vi "FTW-JSON-Object-GetElements-Bool.vi"(0 "JSON Object":refnum<class "FTW-JSON.lvclass">, 5 "Keys":string[](array[string]), 11 "error in":errorcluster) -> (4 "JSON Object out":refnum<class "FTW-JSON.lvclass">, 6 "Values":bool[](array[boolean]), 8 "All Found?":bool, 10 "Which Found?":bool[](array[boolean]), 15 "error out":errorcluster)   [LabVIEW 2013, in "FTW-JSON.lvclass"]
uses:
  FTW-JSON.lvclass
  FTW-JSON.lvclass/FTW-JSON.ctl
  FTW-JSON-Type.ctl
panel:
  # "Inputs"
  # "Outputs"
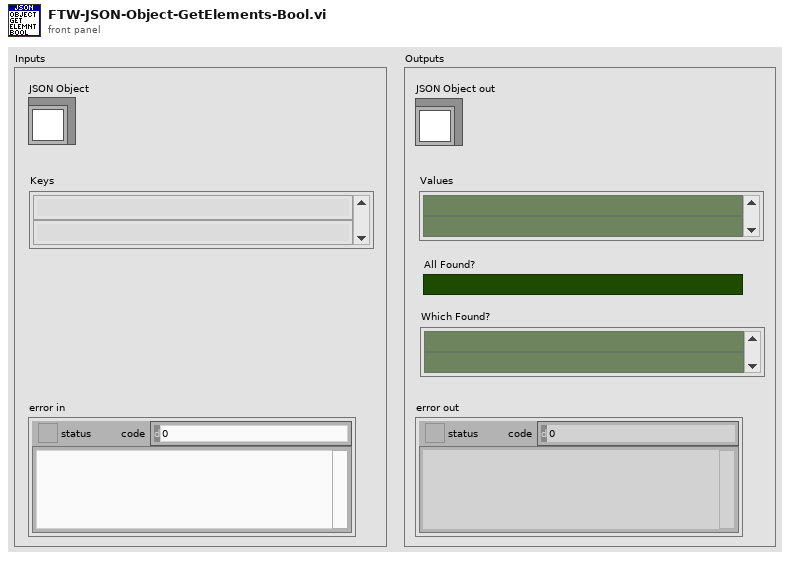
[diagram p1: front panel]
types:
  T1 = typedef "FTW-JSON-Type.ctl" = enum16{"Object", "Array", "String", "Integer", "Floating Point", "true", "false", "null", "undefined"}
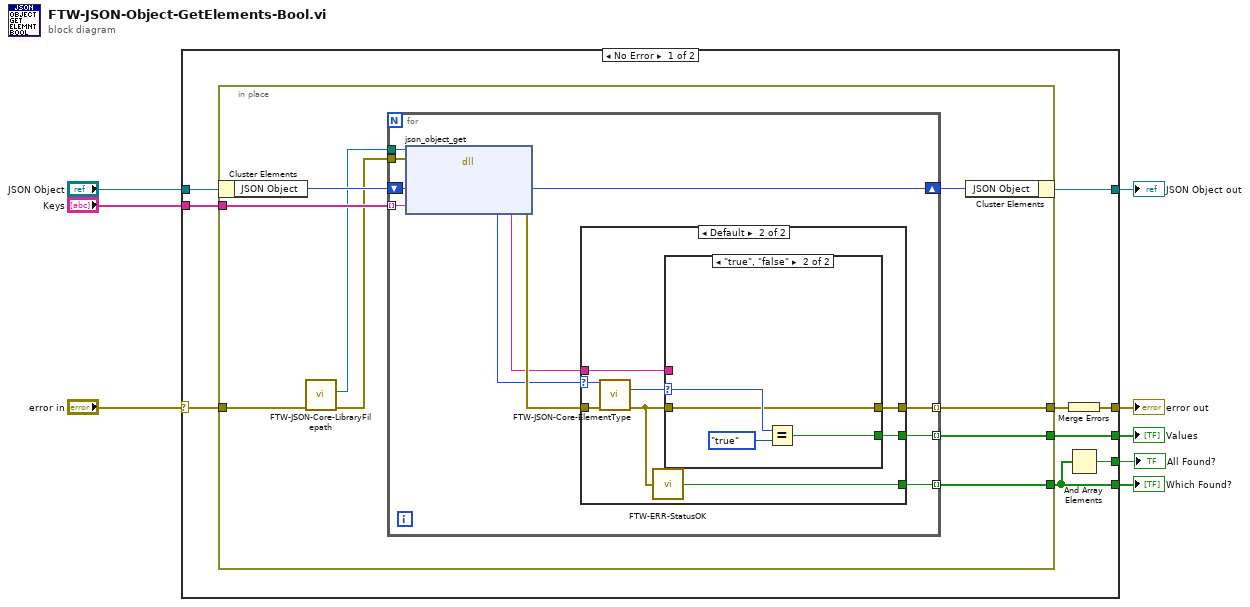
[diagram p0: block diagram]
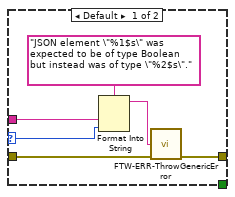
[diagram p3: hidden frame]
diagram:
  n1 = case shown="No Error" "error in" {
    selector: "error in" -> [w17 w58]
    tunnel: [w11 w58] -> w8
    tunnel: [w15 w57] -> w6
    tunnel: "JSON Object" -> [w16 w57]
    tunnel: "Keys" -> [w14 _]
    tunnel: [w12 _] -> w3
    tunnel: [w10 _] -> w2
    tunnel: [w9 _] -> w1
    frame No Error {
      n2 = in-place {
        in-place-border: w17 -> [w26]
        in-place-border: w14 -> [w24]
        in-place-border: [w21] -> w13
        in-place-border: [w20] -> w12
        in-place-border: [w18] -> w10
        n3 = in-place-cluster #1(w16) -> ("JSON Object"=w25:i64)
        n4 = call "FTW-JSON-Core-LibraryFilepath.vi"("error in"=w26) -> ("error out"=w23:errorcluster, "JSON Library Filepath"=w22:path)  [unwired: 9 in]
        n5 = for {
          tunnel: w24 -> [w36] mode=indexing
          tunnel: w23 -> [w35]
          tunnel: w22 -> [w34]
          tunnel: [w32] -> w21 mode=indexing
          tunnel: [w31] -> w20 mode=indexing
          tunnel: [w28] -> w18 mode=indexing
          shift-right: [w29] -> w19
          shift-left: w25 -> [w37]
          n6 = dll-call lib="?" fn="json_object_get"(path in=w34, error in=w35, "JSON Object Pointer"=w37, "Element Key"=w36) -> (error out=w33:errorcluster, "JSON Element Pointer"=w30:i64, "JSON Object Pointer"=w29:i64, "Element Key"=w27:string)  [unwired: 1 in, 1 out]
          n7 = case shown="Default" w30 {
            selector: w30 -> [_ w46]
            tunnel: w33 -> [w38 w42]
            tunnel: [w38 w43] -> w32
            tunnel: [_ w45] -> w31
            tunnel: [_ w40] -> w28
            tunnel: w27 -> [_ w41]
            frame 0 {
            }
            frame Default {
              n8 = call "FTW-JSON-Core-ElementType.vi"("JSON Element"=w46, "error in"=w42) -> ("JSON Type"=w44:T1, "error out"=w39:errorcluster)  [unwired: 11 in, 1 out]
              n9 = call "FTW-ERR-StatusOK.vi"("error to check"=w39) -> ("Status OK?"=w40:bool)
              n10 = case shown="\"true\", \"false\"" w44 {
                selector: w44 -> [w48 w54]
                tunnel: [_ w55] -> w45
                tunnel: w39 -> [w52 w53]
                tunnel: [w47 w53] -> w43
                tunnel: w41 -> [w49 _]
                frame Default {
                  n11 = Format Into String(format string="JSON element \"%1$s\" was expected to be of type Boolean but instead was of type \"%2$s\"." ("Error Message"), w49, w48) -> (resulting string=w50:string)  [unwired: 2 in, 1 out]
                  n12 = call "FTW-ERR-ThrowGenericError.vi"("Error Message"=w50, "error in"=w52) -> ("error out"=w47:errorcluster)  [unwired: 13 in]
                }
                frame "true", "false" {
                  n13 = Equal?(x=w54, y=FTW-JSON-Type."true" ("x")) -> (x = y?=w55:bool)
                }
              }
            }
          }
        }
        n14 = in-place-cluster #1("JSON Object"=w19) -> (w15:refnum<class "FTW-JSON.lvclass">)
      }
      n15 = Merge Errors(w13) -> (w11:errorcluster)
      n16 = And Array Elements(Boolean array=w10) -> (logical AND=w9:bool)
    }
    frame Error {
    }
  }
  "error out" <- w8
  "JSON Object out" <- w6
  "Which Found?" <- w2
  "Values" <- w3
  "All Found?" <- w1
